vi "Mach1-Test-08-16.vi"() -> ()   [LabVIEW 2010]
uses:
  <vilib>/eio/EIONode/EIONode.xnode
  <vilib>/rvi/eio/nirviEIOImplementation/nirviEIOImplementation.xnode
  <vilib>/rvi/eio/common/nirviEmuClasses.ctl
  <vilib>/rvi/eio/common/nirviEmuTemplateMethod_noerrors.vi
panel:
  in  "2Pos1A":bool
  in  "Fan2":bool
  in  "Fan1":bool
  in  "USetp[V]Mach2":fxp<+/-,16,4> format="%.14g"
  in  "USetp[V]Mach1":fxp<+/-,16,4> format="%.14g"
  in  "Umax[V]Mach2":fxp<+/-,16,4> format="%.14g"
  in  "Umax[V]Mach1":fxp<+/-,16,4> format="%.14g"
  in  "PIDMach2":T1 {"proportional gain (Kc)" format="%.11g"; "integral gain (Kc*Ts/Ti)" format="%.11g"; "derivative gain (Kc*Td/Ts)" format="%.11g"}
  in  "PIDMach1":T1 {"proportional gain (Kc)" format="%.11g"; "integral gain (Kc*Ts/Ti)" format="%.11g"; "derivative gain (Kc*Td/Ts)" format="%.11g"}
  in  "Heizen?Mach2":bool
  in  "Heizen?Mach1":bool
  out "U[V]Mach1":fxp<+/-,16,4> format="%.25g"
  out "U[V]Mach2":fxp<+/-,16,4> format="%.25g"
  in  "Abstand zwischen Messungen [us]Mach":u16 caption="Abstand zwischen Messungen Mach [us]"
  in  "wie viele Messwerte?Mach":u16
  in  "vor der Messung [us]Mach":u16=200
  in  "Per[us]Mach":u16 caption="Periode Mach [us]"
  in  "stop":bool
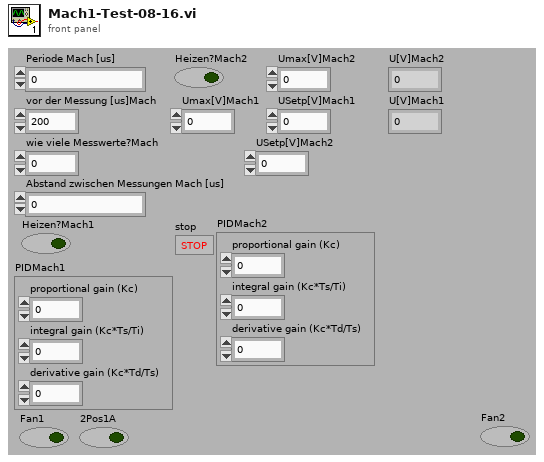
[diagram p1: front panel]
types:
  T1 = cluster{"proportional gain (Kc)":fxp<+/-,16,8>, "integral gain (Kc*Ts/Ti)":fxp<+/-,16,8>, "derivative gain (Kc*Td/Ts)":fxp<+/-,16,8>}
  T2 = typedef "nirviEmuClasses.ctl" = enum16{"IO Read", "IO Write", "Method", "Property Read", "Property Write"}
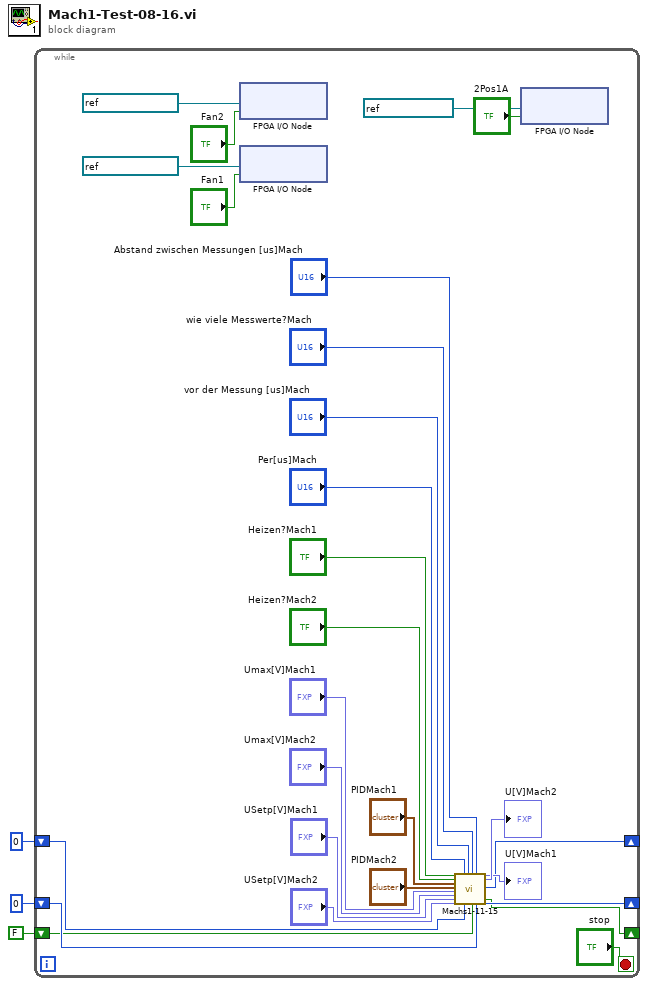
[diagram p0: block diagram]
diagram:
  n1 = while {
    shift-right: [w15] -> _
    shift-left: u16 0 ("Mach1maxHigh") -> [w14]
    shift-right: [w13] -> _
    shift-left: u16 0 ("Mach2High") -> [w12]
    shift-right: [w11] -> _
    shift-left: FALSE ("Mach2High?") -> [w10]
    stop <- "stop" stop-if-true
    n2 = xnode "FPGA I/O Node"("I/O Item"="Fan2", "FPGA I/O In"=refnum<k21> "Mod6/DIO31") -> ()  [unwired: 1 out]
    n3 = xnode "FPGA I/O Node"("I/O Item"="Fan1", "FPGA I/O In"=refnum<k21> "Mod6/DIO30") -> ()  [unwired: 1 out]
    n4 = call "Machs1-11-15.vi"("Heizen?Mach1"="Heizen?Mach1", "Heizen?Mach2"="Heizen?Mach2", "PIDMach1"="PIDMach1", "PIDMach2"="PIDMach2", "Umax[V]Mach1"="Umax[V]Mach1", "Umax[V]Mach2"="Umax[V]Mach2", "USetp[V]Mach1"="USetp[V]Mach1", "USetp[V]Mach2"="USetp[V]Mach2", "Per[us]Mach"="Per[us]Mach", "Mach1maxHigh"=w14, "vor der Messung [us]Mach"="vor der Messung [us]Mach", "wie viele Messwerte?Mach"="wie viele Messwerte?Mach", "Mach2High?"=w10, "Abstand zwischen Messungen [us]Mach"="Abstand zwischen Messungen [us]Mach", "Mach2High"=w12) -> ("U[V]Mach1"=→"U[V]Mach1":fxp<+/-,16,4>, "U[V]Mach2"=→"U[V]Mach2":fxp<+/-,16,4>, "Mach1maxHigh"=w15:u16, "Mach2High?"=w11:bool, "Mach2High"=w13:u16)  [unwired: 8 in]
    n5 = xnode "FPGA I/O Node"("I/O Item"="2Pos1A", "FPGA I/O In"=refnum<k21> "Mod6/DIO6") -> ()  [unwired: 1 out]
  }
